vi "OE2052_Configure Auto_Setting.vi"(7 "OE2052_Auto Setting":T1={"Auto Range"=FALSE, "Auto Offest"=FALSE, "Auto Phase"=FALSE, "channel"=1, "Demod channel(phase)"=1} {"Demod channel(phase)" items=["Demod 1"=1, "Demod 2"=2, "Demod 3"=3, "Demod 4"=4]; "channel" items=["A"=1, "B"=2]}, 8 "Error in (no error)":errorcluster caption="error out（no error）", 9 "Remote Mode":u16(ring) items=["USB"=0, "RS232"=1, "Ethernet"=3], 10 "Connection ID in":refnum<k5>, 11 "VISA resource name":refnum<visa-resource-name>) -> (0 "Error out":errorcluster caption="error out", 1 "Output String":string, 2 "Connection ID out":refnum<k5>, 3 "VISA resource  out":refnum<visa-resource-name>)   [LabVIEW 2011]
panel:
  out "Demod channel(phase)":u16
  out "channel":u16
  out "字符串":string
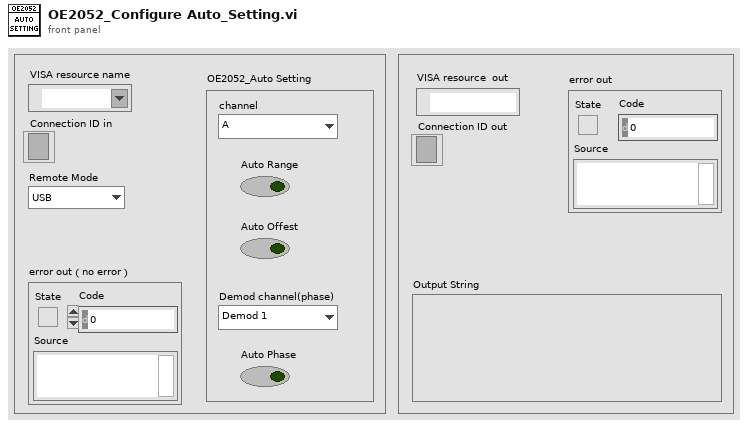
[diagram p1: front panel]
types:
  T1 = cluster{"Auto Range":bool, "Auto Offest":bool, "Auto Phase":bool, "channel":u16, "Demod channel(phase)":u16}
  T2 = cluster{bool, bool, bool, "channel":u16, "Demod channel(phase)":u16}
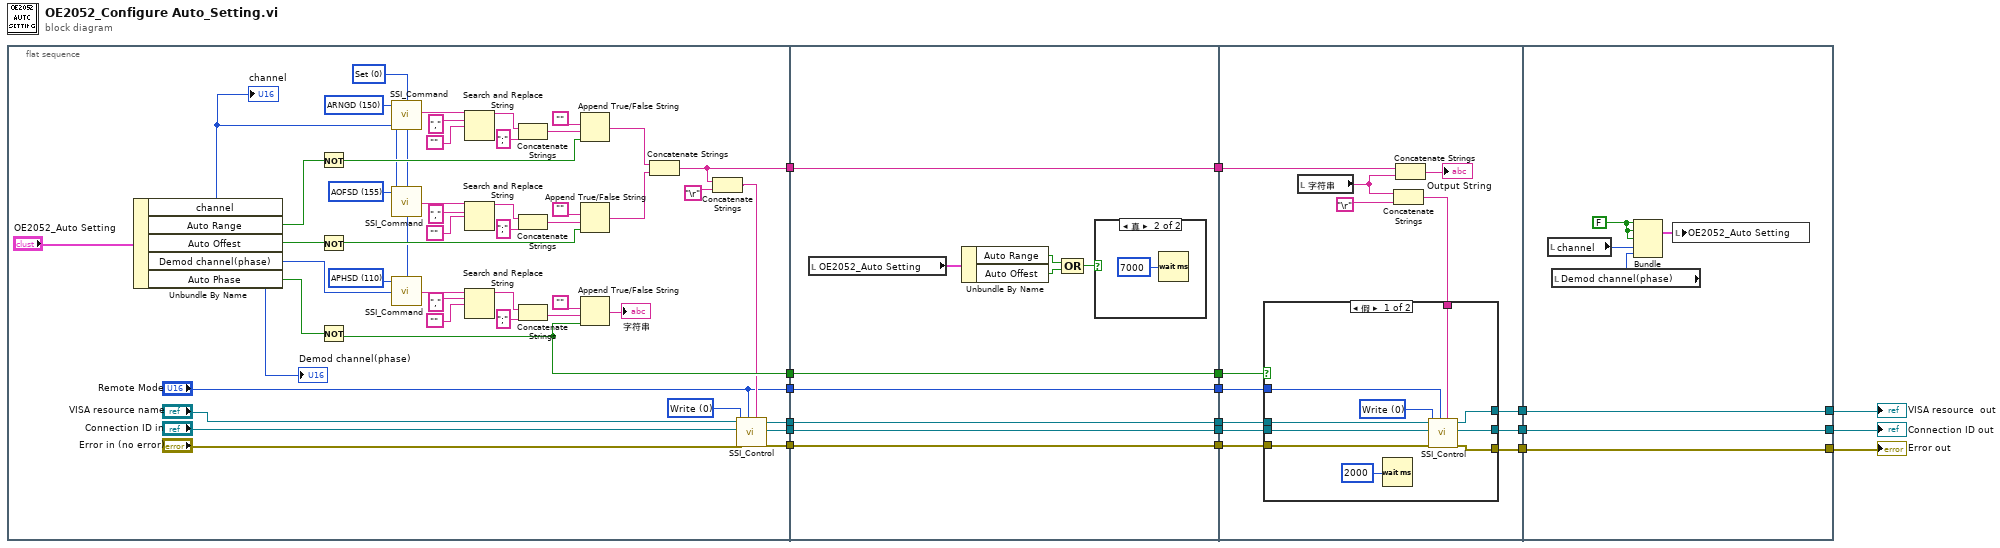
[diagram p0: block diagram]
diagram:
  n1 = flat-sequence {
    tunnel: [w62] -> w18
    tunnel: [w61] -> w17
    tunnel: [w60] -> w16
    tunnel: [w32] -> w11
    tunnel: [w27] -> w7
    tunnel: ["Remote Mode"] -> w5
    tunnel: w18 -> [w76]
    tunnel: w17 -> [w75]
    tunnel: w16 -> [w74]
    tunnel: [w76] -> w15
    tunnel: [w75] -> w14
    tunnel: [w74] -> w13
    tunnel: [w69] -> w12
    tunnel: w11 -> [w69]
    tunnel: w7 -> [w68]
    tunnel: [w68] -> w6
    tunnel: w5 -> [w67]
    tunnel: [w67] -> w4
    tunnel: w15 -> [w88]
    tunnel: w14 -> [w89]
    tunnel: w13 -> [w87]
    tunnel: w12 -> [w90]
    tunnel: w6 -> [w82]
    tunnel: w4 -> [w81]
    tunnel: [w86] -> w3
    tunnel: [w85] -> w2
    tunnel: [w84] -> w1
    tunnel: [w108] -> w8
    tunnel: [w109] -> w9
    tunnel: [w110] -> w10
    tunnel: w3 -> [w110]
    tunnel: w2 -> [w109]
    tunnel: w1 -> [w108]
    frame #0 {
      w22 = u16 110 items=["ISRC", "IGND", "ICPL", "ILIN", "PHAS", "FMOD", "RSLP", "FREQ", "SWPT", "SLLM", "SULM", "SSLL", "SSLG", "STLM", "SWRM", "IRNG", "SENS", "RMOD", "OFLT", "OFSL", "SYNC", "DMOD", "HARM", "DARB", "SWVT", "SLVL", "SVLL", "SVUL", "SVSL", "SVSG", "SVTM", "SVRM", "RALL", "SNAP", "OUTP", "OAUX", "COUT", "CAUX", "COFP", "CEXP", "FPOP", "OEXP", "*IDN", "*RST", "OVLD", "INOV", "GNOV", "*PLL", "SSET", "RSET", "AGAN", "APHS", "ARSV", "ASCL", "EQCD", "EQCS", "SPED", "SRAT", "SLEN", "SSLE", "STRG", "SPRM", "STRD", "PAUS", "REST", "SPTS", "TRCA", "TEMP", "RSTU", "INHZ", "DEQU", "SADD", "ARNG", "CSPE", "ISRCD", "IGNDD", "ICPLD", "ILIND", "PHASD", "FMODD", "RSLPD", "FREQD", "SWPTD", "SLLMD", "SULMD", "SSLLD", "SSLGD", "STLMD", "SWRMD", "SENSD", "RMODD", "OFLTD", "OFSLD", "SYNCD", "HARMD", "EQCDD", "EQCSD", "SNAPD", "OUTPD", "SWVTD", "SLVLD", "SVLLD", "SVULD", "SVSLD", "SVSGD", "SVTMD", "SVRMD", "SVDCD", "ARSVD", "AGAND", "APHSD", "ASCLD", "FPOPD", "CAUXD", "OEXPD", "SPEDD", "SRATD", "SLEND", "SSLED", "STRGD", "SPRMD", "STRDD", "PAUSD", "RESTD", "SPTSD", "TRCAD", "*IDND", "*RSTD", "INOVD", "GNOVD", "*PLLD", "SSETD", "RSETD", "RALLD", "NIPA", "NSMA", "NGWA", "NMAC", "NMOD", "TRIG", "TRCB", "INHZD", "ISAMD", "IRAGD", "RRAGD", "SOFFD", "DMODD", "COUTD", "COFPD", "CEXPD", "ARNGD", "OAUXD", "TRIM", "SUITD", "SNHZD", "AOFSD"] ("Command Type")
      w23 = u16 155 items=["ISRC", "IGND", "ICPL", "ILIN", "PHAS", "FMOD", "RSLP", "FREQ", "SWPT", "SLLM", "SULM", "SSLL", "SSLG", "STLM", "SWRM", "IRNG", "SENS", "RMOD", "OFLT", "OFSL", "SYNC", "DMOD", "HARM", "DARB", "SWVT", "SLVL", "SVLL", "SVUL", "SVSL", "SVSG", "SVTM", "SVRM", "RALL", "SNAP", "OUTP", "OAUX", "COUT", "CAUX", "COFP", "CEXP", "FPOP", "OEXP", "*IDN", "*RST", "OVLD", "INOV", "GNOV", "*PLL", "SSET", "RSET", "AGAN", "APHS", "ARSV", "ASCL", "EQCD", "EQCS", "SPED", "SRAT", "SLEN", "SSLE", "STRG", "SPRM", "STRD", "PAUS", "REST", "SPTS", "TRCA", "TEMP", "RSTU", "INHZ", "DEQU", "SADD", "ARNG", "CSPE", "ISRCD", "IGNDD", "ICPLD", "ILIND", "PHASD", "FMODD", "RSLPD", "FREQD", "SWPTD", "SLLMD", "SULMD", "SSLLD", "SSLGD", "STLMD", "SWRMD", "SENSD", "RMODD", "OFLTD", "OFSLD", "SYNCD", "HARMD", "EQCDD", "EQCSD", "SNAPD", "OUTPD", "SWVTD", "SLVLD", "SVLLD", "SVULD", "SVSLD", "SVSGD", "SVTMD", "SVRMD", "SVDCD", "ARSVD", "AGAND", "APHSD", "ASCLD", "FPOPD", "CAUXD", "OEXPD", "SPEDD", "SRATD", "SLEND", "SSLED", "STRGD", "SPRMD", "STRDD", "PAUSD", "RESTD", "SPTSD", "TRCAD", "*IDND", "*RSTD", "INOVD", "GNOVD", "*PLLD", "SSETD", "RSETD", "RALLD", "NIPA", "NSMA", "NGWA", "NMAC", "NMOD", "TRIG", "TRCB", "INHZD", "ISAMD", "IRAGD", "RRAGD", "SOFFD", "DMODD", "COUTD", "COFPD", "CEXPD", "ARNGD", "OAUXD", "TRIM", "SUITD", "SNHZD", "AOFSD"] ("Command Type")
      w25 = u16 150 items=["ISRC", "IGND", "ICPL", "ILIN", "PHAS", "FMOD", "RSLP", "FREQ", "SWPT", "SLLM", "SULM", "SSLL", "SSLG", "STLM", "SWRM", "IRNG", "SENS", "RMOD", "OFLT", "OFSL", "SYNC", "DMOD", "HARM", "DARB", "SWVT", "SLVL", "SVLL", "SVUL", "SVSL", "SVSG", "SVTM", "SVRM", "RALL", "SNAP", "OUTP", "OAUX", "COUT", "CAUX", "COFP", "CEXP", "FPOP", "OEXP", "*IDN", "*RST", "OVLD", "INOV", "GNOV", "*PLL", "SSET", "RSET", "AGAN", "APHS", "ARSV", "ASCL", "EQCD", "EQCS", "SPED", "SRAT", "SLEN", "SSLE", "STRG", "SPRM", "STRD", "PAUS", "REST", "SPTS", "TRCA", "TEMP", "RSTU", "INHZ", "DEQU", "SADD", "ARNG", "CSPE", "ISRCD", "IGNDD", "ICPLD", "ILIND", "PHASD", "FMODD", "RSLPD", "FREQD", "SWPTD", "SLLMD", "SULMD", "SSLLD", "SSLGD", "STLMD", "SWRMD", "SENSD", "RMODD", "OFLTD", "OFSLD", "SYNCD", "HARMD", "EQCDD", "EQCSD", "SNAPD", "OUTPD", "SWVTD", "SLVLD", "SVLLD", "SVULD", "SVSLD", "SVSGD", "SVTMD", "SVRMD", "SVDCD", "ARSVD", "AGAND", "APHSD", "ASCLD", "FPOPD", "CAUXD", "OEXPD", "SPEDD", "SRATD", "SLEND", "SSLED", "STRGD", "SPRMD", "STRDD", "PAUSD", "RESTD", "SPTSD", "TRCAD", "*IDND", "*RSTD", "INOVD", "GNOVD", "*PLLD", "SSETD", "RSETD", "RALLD", "NIPA", "NSMA", "NGWA", "NMAC", "NMOD", "TRIG", "TRCB", "INHZD", "ISAMD", "IRAGD", "RRAGD", "SOFFD", "DMODD", "COUTD", "COFPD", "CEXPD", "ARNGD", "OAUXD", "TRIM", "SUITD", "SNHZD", "AOFSD"] ("Command Type")
      w24 = u16 0 items=["Set", "Query"] ("Opera")
      w63 = u16 0 items=["Write", "Read"] ("Control")
      n2 = Unbundle By Name("OE2052_Auto Setting") -> ("channel"=w21:u16, "Auto Range"=w33:bool, "Auto Offest"=w36:bool, "Demod channel(phase)"=w19:u16, "Auto Phase"=w20:bool)
      "channel" <- w21
      "Demod channel(phase)" <- w19
      n3 = Not(x=w33) -> (.not. x?=w34:bool)
      n4 = Not(x=w36) -> (.not. x?=w35:bool)
      n5 = Not(x=w20) -> (.not. x?=w32:bool)
      n6 = call "SSI_Command.vi"("Opera"=w24, "channel"=w21, "Command Type"=w25) -> ("Output string"=w39:string)  [unwired: 1 in]
      n7 = call "SSI_Command.vi"("Opera"=w24, "channel"=w21, "Command Type"=w23) -> ("Output string"=w41:string)  [unwired: 1 in]
      n8 = call "SSI_Command.vi"("Opera"=w24, "channel"=w19, "Command Type"=w22) -> ("Output string"=w40:string)  [unwired: 1 in]
      n9 = Search and Replace String(input string=w39, search string="," ("搜索字符串"), replace string="") -> (result string=w51:string)  [unwired: 5 in, 3 out]
      n10 = Search and Replace String(input string=w41, search string="," ("搜索字符串"), replace string="") -> (result string=w48:string)  [unwired: 5 in, 3 out]
      n11 = Search and Replace String(input string=w40, search string="," ("搜索字符串"), replace string="") -> (result string=w45:string)  [unwired: 5 in, 3 out]
      n12 = Concatenate Strings(w51, ";") -> (w44:string)
      n13 = Concatenate Strings(w48, ";") -> (w43:string)
      n14 = Concatenate Strings(w45, ";") -> (w42:string)
      n15 = Append True/False String(1:w34, 2:w44, 3:"") -> (0:w31:string)  [unwired: 1 in]
      n16 = Append True/False String(1:w35, 2:w43, 3:"") -> (0:w30:string)  [unwired: 1 in]
      n17 = Append True/False String(1:w32, 2:w42, 3:"") -> (0:→"字符串":string)  [unwired: 1 in]
      n18 = Concatenate Strings(w31, w30) -> (w27:string)
      n19 = Concatenate Strings(w27, "\r") -> (w28:string)
      n20 = call "SSI_Control.vi"("Write Buffer"=w28, "Remote Mode"="Remote Mode", "Error in (no error)"="Error in (no error)", "Control"=w63, "Connection ID in"="Connection ID in", "VISA resource name"="VISA resource name") -> ("Error out"=w60:errorcluster, "Connection ID out"=w62:refnum<k5>, "VISA resource  out"=w61:refnum<visa-resource-name>)  [unwired: 2 in, 1 out]
    }
    frame #1 {
      n21 = local read "OE2052_Auto Setting"() -> (w70:T1)
      n22 = Unbundle By Name(w70) -> ("Auto Range"=w72:bool, "Auto Offest"=w71:bool)
      n23 = Compound Arithmetic op=OR(w72, w71) -> (w73:bool)
      n24 = case shown="真" w73 {
        frame False {
        }
        frame True {
          n25 = Wait (ms)(milliseconds to wait=u32 7000 ("等待时间（毫秒）")) -> ()  [unwired: 1 out]
        }
      }
    }
    frame #2 {
      n26 = local read "字符串"() -> (w80:string)
      n27 = Concatenate Strings(w80, "\r") -> (w78:string)
      n28 = case shown="假" w90 {
        tunnel: w89 -> [w99 w103]
        tunnel: w88 -> [w98 w102]
        tunnel: w87 -> [w97 w101]
        tunnel: [w96 w101] -> w86
        tunnel: [w95 w102] -> w85
        tunnel: [w94 w103] -> w84
        tunnel: w78 -> [w92 _]
        tunnel: w81 -> [w91 _]
        frame False {
          w100 = u16 0 items=["Write", "Read"] ("Control")
          n29 = Wait (ms)(milliseconds to wait=u32 2000 ("等待时间（毫秒）")) -> ()  [unwired: 1 out]
          n30 = call "SSI_Control.vi"("Write Buffer"=w92, "Remote Mode"=w91, "Error in (no error)"=w97, "Control"=w100, "Connection ID in"=w98, "VISA resource name"=w99) -> ("Error out"=w96:errorcluster, "Connection ID out"=w95:refnum<k5>, "VISA resource  out"=w94:refnum<visa-resource-name>)  [unwired: 2 in, 1 out]
        }
        frame True {
        }
      }
      n31 = Concatenate Strings(w82, w80) -> (→"Output String":string)
    }
    frame #3 {
      w105 = FALSE
      n32 = local read "channel"() -> (w106:u16)
      n33 = local read "Demod channel(phase)"() -> (w104:u16)
      n34 = Bundle(w105, w105, w105, "channel"=w106, "Demod channel(phase)"=w104) -> (w107:T2)  [unwired: 1 in]
      n35 = local write "OE2052_Auto Setting"(w107) -> ()
    }
  }
  "Error out" <- w10
  "Connection ID out" <- w9
  "VISA resource  out" <- w8
